vi "Add Parameter.vi"(8 "error in":errorcluster, 9 "parameter encoding":T1={"start index"=0, "size"=8, "encoding"=enum."BCD", "signed"=FALSE, "scale multiplier"=1.0, "scale offset"=0.0}, 10 "parameter definition":T4, 11 "label in":T3 format="%.0x") -> (0 "error out":errorcluster, 2 "parameter":T3 format="%.0x", 3 "label out":T3 format="%.0x")   [LabVIEW 2020, in "AIM ARINC 429 Scripting.lvlib"]
doc: "Adds the specified <b>parameter definition</b> with <b>parameter encoding</b> to the system definition in the 'Word' subsection of <b>label in</b>. Returns the newly added <b>parameter</b> reference."
uses:
  AIM ARINC 429 Scripting.lvlib
  Constants.vi
  <vilib>/NI VeriStand/Custom Device API/Custom Device API.lvlib
  <vilib>/NI VeriStand/Custom Device API/Custom Device Channel Type.ctl
  <vilib>/NI VeriStand/Custom Device API/Custom Device Channel.ctl
  <vilib>/NI VeriStand/Custom Device API/Custom Device Item Ref.ctl
  <vilib>/NI/NI VeriStand Encoding and Decoding/Encoding.ctl
  <vilib>/NI/NI VeriStand Encoding and Decoding/Encoding and Decoding.lvlib
  Shared/Parameter Definition.ctl
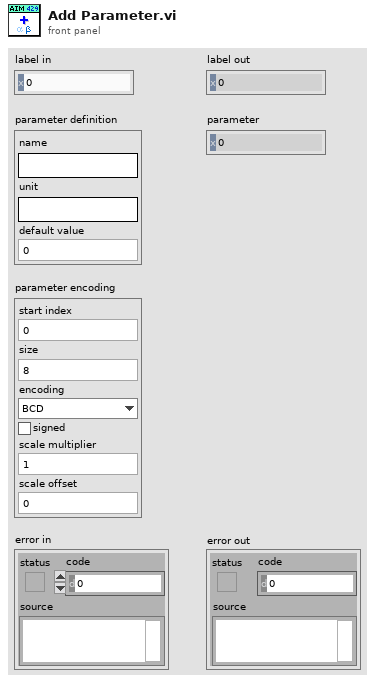
[diagram p1: front panel]
types:
  T1 = typedef "Parameter Definition.ctl" = cluster{"start index":i32, "size":i32, "encoding":T2, "signed":bool, "scale multiplier":dbl, "scale offset":dbl}
  T2 = typedef "Encoding and Decoding.lvlib/Encoding.ctl" = enum16{"BNR", "BCD", "Discrete"}
  T3 = typedef "Custom Device API.lvlib/Custom Device Item Ref.ctl" = u64
  T4 = cluster{"name":string, "unit":string, "default value":dbl}
  T5 = typedef "Custom Device API.lvlib/Custom Device Channel.ctl" = cluster{"Type":T6, "Units":string, "Default Value":dbl, "Faultable":bool, "Scalable":bool}
  T6 = typedef "Custom Device API.lvlib/Custom Device Channel Type.ctl" = enum16{"Input", "Output"}
  T7 = typedef "Direction.ctl" = enum16{"Rx", "Tx"}
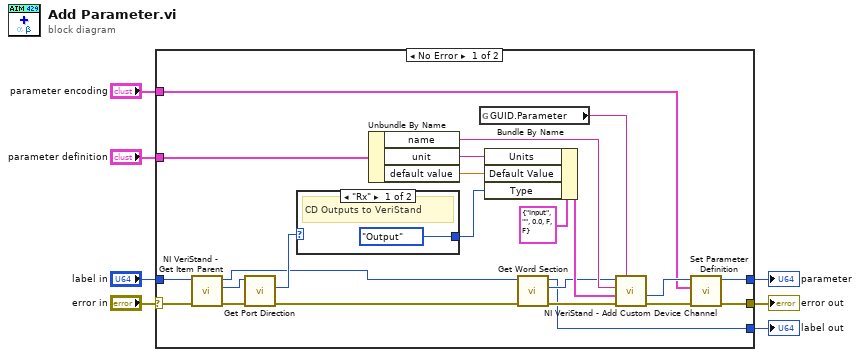
[diagram p0: block diagram]
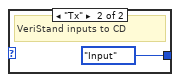
[diagram p2: hidden frame]
diagram:
  n1 = case shown="No Error" "error in" {
    selector: "error in" -> [w19 w34]
    tunnel: [w21 w34] -> w6
    tunnel: "label in" -> [w18 w33]
    tunnel: [w22 _] -> w4
    tunnel: "parameter definition" -> [w26 _]
    tunnel: [w8 w33] -> w2
    tunnel: "parameter encoding" -> [w10 _]
    frame No Error {
      n2 = call <vilib>:"NI VeriStand - Get Item Parent.vi"("error in (no error)"=w19, "Item Ref in"=w18) -> ("error out"=w17:errorcluster, "Parent Ref"=w12:T3, "Item Ref out"=w11:T3)  [unwired: 6 in, 1 out]
      n3 = call "Get Port Direction.vi"("error in"=w17, "port ref in"=w12) -> ("error out"=w16:errorcluster, "direction"=w15:T7)  [unwired: 7 in, 1 out]
      n4 = case shown="\"Rx\"" w15 {
        tunnel: [Custom_Device_Channel_Type."Output" ("Type") Custom_Device_Channel_Type."Input" ("Type")] -> w14
        frame "Rx" {
          # "CD Outputs to VeriStand"
        }
        frame "Tx" {
          # "VeriStand inputs to CD"
        }
      }
      n5 = Unbundle By Name(w26) -> ("name"=w13:string, "unit"=w27:string, "default value"=w25:dbl)
      n6 = global read "Constants.vi" "GUID.Parameter"() -> (w30:string)
      n7 = Bundle By Name(cluster=T5 {"Type"=enum."Input", "Units"="", "Default Value"=0.0, "Faultable"=FALSE, "Scalable"=FALSE} ("Channel"), "Units"=w27, "Default Value"=w25, "Type"=w14) -> (w28:T5)
      n8 = call "Get Word Section.vi"("error in"=w16, "label ref"=w11) -> ("error out"=w20:errorcluster, "word ref"=w9:T3, "label ref out"=w8:T3)  [unwired: 7 in]
      n9 = call <vilib>:"NI VeriStand - Add Custom Device Channel.vi"("GUID (Default Channel)"=w30, "error in (no error)"=w20, "Channel"=w28, "Channel Name"=w13, "Parent Ref in"=w9) -> ("error out"=w24:errorcluster, "Channel Ref"=w23:T3)  [unwired: 3 in, 2 out]
      n10 = call "Set Parameter Definition.vi"("error in"=w24, "parameter definition"=w10, "parameter ref in"=w23) -> ("error out"=w21:errorcluster, "parameter ref out"=w22:T3)  [unwired: 7 in]
    }
    frame Error {
    }
  }
  "parameter" <- w4
  "error out" <- w6
  "label out" <- w2
